vi "DAQmx Create Virtual Channel (CI Frequency).vi"(0 "task in":refnum<class "Session Factory.lvclass">, 1 "maximum value":dbl=100.0 format="%0.6f", 2 "minimum value":dbl=2.0 format="%0.6f", 3 "measurement method":i32(ring)=10105 items=["Low Frequency with 1 Counter"=10105, "High Frequency with 2 Counters"=10157, "Large Range with 2 Counters"=10205, "Dynamic Averaging"=16065], 5 "counter":tag, 6 "divisor":u32=4, 7 "name to assign":string, 9 "units":i32(ring)=10373 items=["Hz"=10373, "Ticks"=10304, "From Custom Scale"=10065], 11 "error in":errorcluster, 12 "custom scale name":tag, 13 "starting edge":i32(ring)=10280 items=["Rising"=10280, "Falling"=10171], 14 "measurement time":dbl=0.001 format="%0.6f") -> (4 "task out":refnum<class "Session Factory.lvclass">, 15 "error out":errorcluster)   [LabVIEW 2021, in "Session Management niDAQmx.lvlib" / "Session Factory.lvclass"]
doc: "Creates a channel to measure the frequency of a digital signal. With the exception of devices that support multi-counter tasks, you can create only one counter input channel at a time with this VI because a task can contain only one counter input channel. To read from multiple counters simultaneously, use a separate task for each counter. Connect the input signal to the default input terminal of the counter unless you select a different input terminal."
uses:
  Session Factory.lvclass
  NI_DAQmx_client/RPC Messages/nidaqmx_grpc_CreateCIFreqChanRequest.ctl
  NI_DAQmx_client/RPC Messages/nidevice_grpc_Session.ctl
  NI_DAQmx_client/RPC Messages/nidevice_grpc_Session_session/nidevice_grpc_Session_session.lvclass
  NI_DAQmx_client/RPC Messages/nidaqmx_grpc_CreateCIFreqChanRequest_units_enum/nidaqmx_grpc_CreateCIFreqChanRequest_units_enum.lvclass
  NI_DAQmx_client/RPC Messages/nidaqmx_grpc_CreateCIFreqChanRequest_edge_enum/nidaqmx_grpc_CreateCIFreqChanRequest_edge_enum.lvclass
  NI_DAQmx_client/RPC Messages/nidaqmx_grpc_CreateCIFreqChanRequest_meas_method_enum/nidaqmx_grpc_CreateCIFreqChanRequest_meas_method_enum.lvclass
  Session Factory.lvclass/Session Factory.ctl
  NI_DAQmx_client/RPC Messages/nidaqmx_grpc_CounterFrequencyMethod.ctl
  NI_DAQmx_client/RPC Messages/nidaqmx_grpc_CreateCIFreqChanRequest_meas_method_enum/nidaqmx_grpc_CreateCIFreqChanRequest_meas_method_enum.lvclass/nidaqmx_grpc_CreateCIFreqChanRequest_meas_method_enum.ctl
  NI_DAQmx_client/RPC Messages/nidaqmx_grpc_FrequencyUnits3.ctl
  NI_DAQmx_client/RPC Messages/nidaqmx_grpc_CreateCIFreqChanRequest_units_enum/nidaqmx_grpc_CreateCIFreqChanRequest_units_enum.lvclass/nidaqmx_grpc_CreateCIFreqChanRequest_units_enum.ctl
  NI_DAQmx_client/RPC Messages/nidaqmx_grpc_Edge1.ctl
  NI_DAQmx_client/RPC Messages/nidaqmx_grpc_CreateCIFreqChanRequest_edge_enum/nidaqmx_grpc_CreateCIFreqChanRequest_edge_enum.lvclass/nidaqmx_grpc_CreateCIFreqChanRequest_edge_enum.ctl
  NI_DAQmx_client/NI_DAQmx_client.lvlib
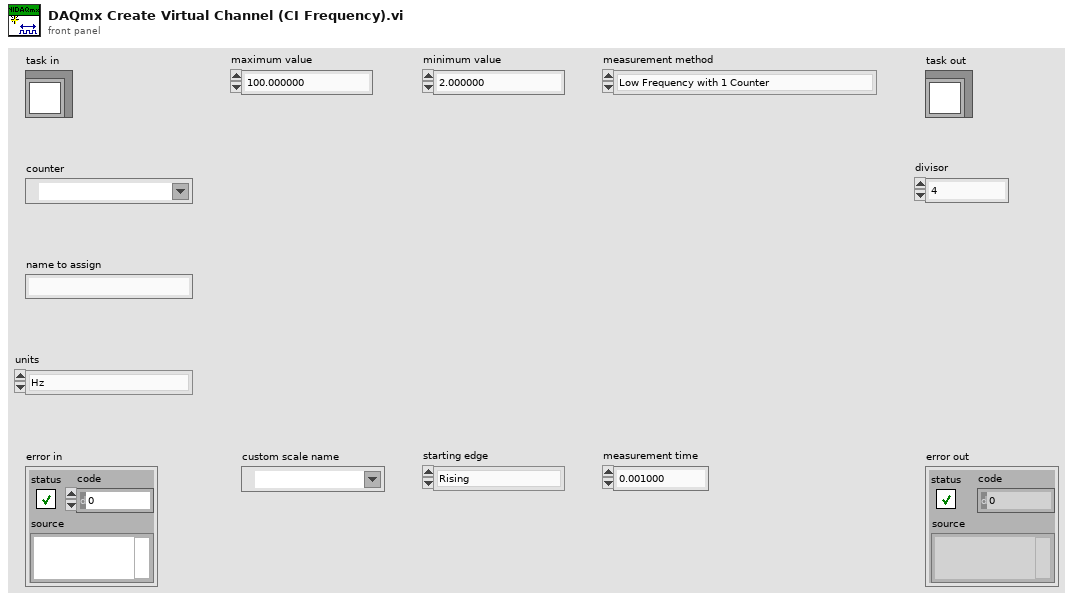
[diagram p1: front panel]
types:
  T1 = typedef "NI_DAQmx_client.lvlib/nidaqmx_grpc_CreateCIFreqChanRequest.ctl" = cluster{"task":T2, "counter":string, "name_to_assign_to_channel":string, "min_val":dbl, "max_val":dbl, "nidaqmx_grpc_CreateCIFreqChanRequest_units_enum":refnum<class "nidaqmx_grpc_CreateCIFreqChanRequest_units_enum.lvclass">, "nidaqmx_grpc_CreateCIFreqChanRequest_edge_enum":refnum<class "nidaqmx_grpc_CreateCIFreqChanRequest_edge_enum.lvclass">, "nidaqmx_grpc_CreateCIFreqChanRequest_meas_method_enum":refnum<class "nidaqmx_grpc_CreateCIFreqChanRequest_meas_method_enum.lvclass">, "meas_time":dbl, "divisor":u32, "custom_scale_name":string}
  T2 = typedef "NI_DAQmx_client.lvlib/nidevice_grpc_Session.ctl" = cluster{"nidevice_grpc_Session_session":refnum<class "nidevice_grpc_Session_session.lvclass">}
  T3 = typedef "NI_DAQmx_client.lvlib/nidaqmx_grpc_Edge1.ctl" = enum32{"EDGE1_UNSPECIFIED", "EDGE1_RISING", "EDGE1_FALLING"}
  T4 = typedef "NI_DAQmx_client.lvlib/nidaqmx_grpc_FrequencyUnits3.ctl" = enum32{"FREQUENCY_UNITS3_UNSPECIFIED", "FREQUENCY_UNITS3_HZ", "FREQUENCY_UNITS3_TICKS", "FREQUENCY_UNITS3_FROM_CUSTOM_SCALE"}
  T5 = typedef "NI_DAQmx_client.lvlib/nidaqmx_grpc_CounterFrequencyMethod.ctl" = enum32{"COUNTER_FREQUENCY_METHOD_UNSPECIFIED", "COUNTER_FREQUENCY_METHOD_LOW_FREQ_1_CTR", "COUNTER_FREQUENCY_METHOD_HIGH_FREQ_2_CTR", "COUNTER_FREQUENCY_METHOD_LARGE_RNG_2_CTR", "COUNTER_FREQUENCY_METHOD_DYN_AVG"}
  T6 = typedef "grpc-lvsupport-release.lvlib/grpcId.ctl" = u64
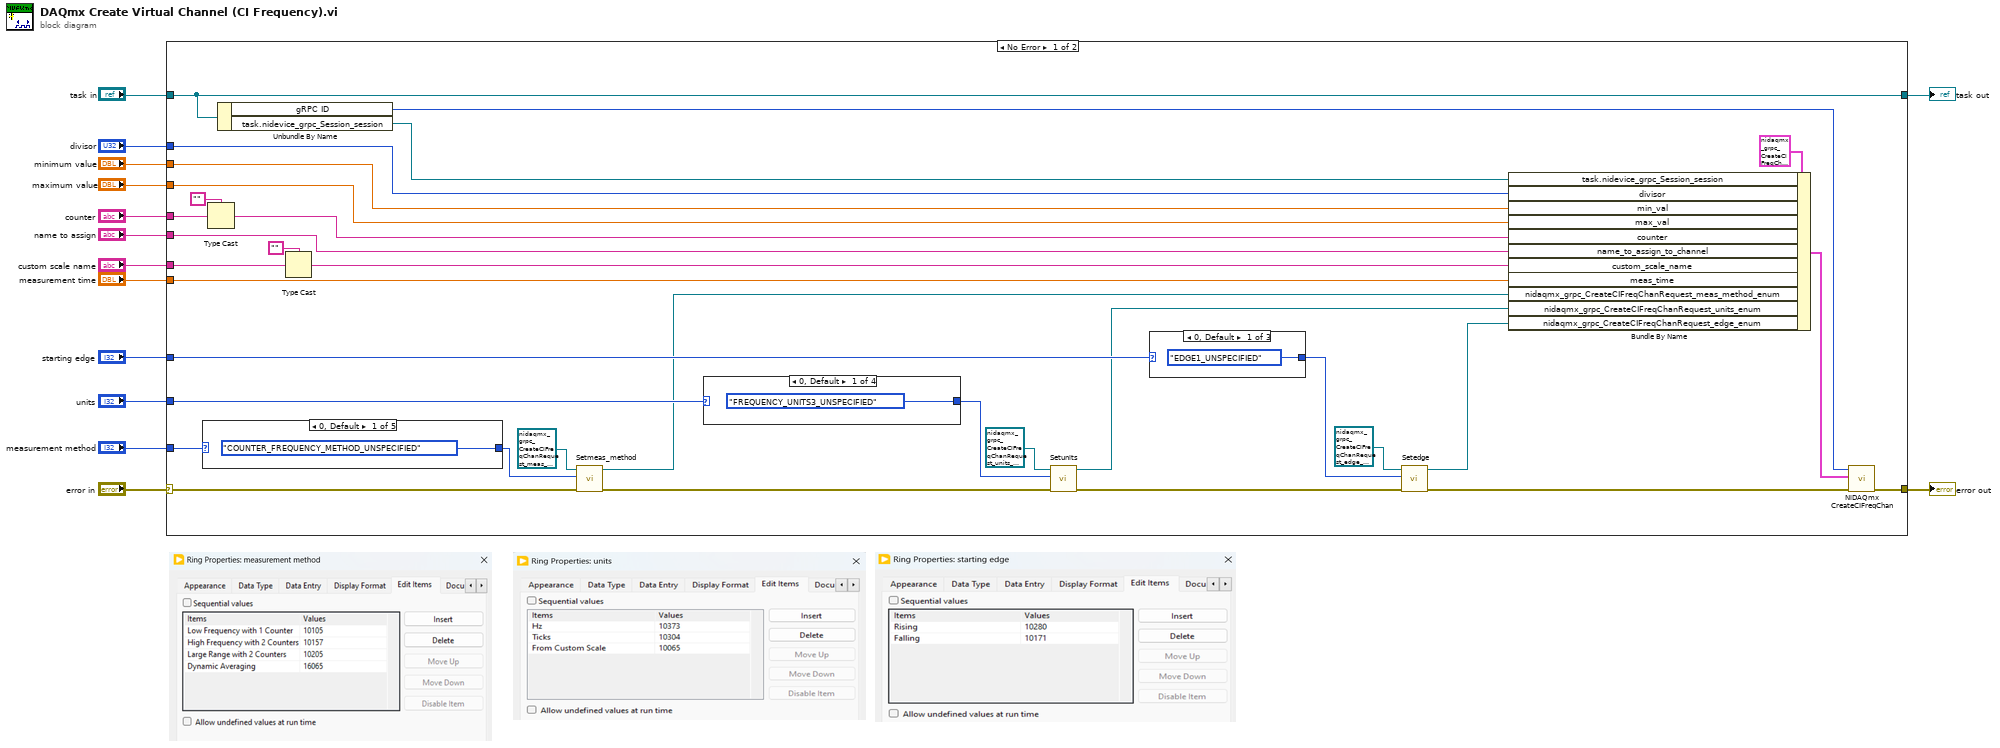
[diagram p0: block diagram]
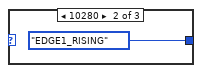
[diagram p2: hidden frame]
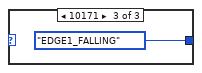
[diagram p3: hidden frame]
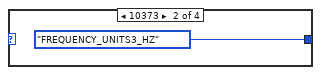
[diagram p4: hidden frame]
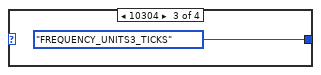
[diagram p5: hidden frame]
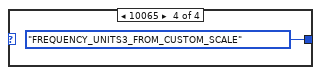
[diagram p6: hidden frame]
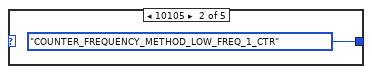
[diagram p7: hidden frame]
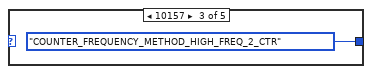
[diagram p8: hidden frame]
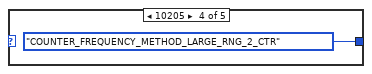
[diagram p9: hidden frame]
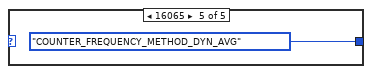
[diagram p10: hidden frame]
diagram:
  n1 = case shown="No Error" "error in" {
    selector: "error in" -> [w40 w61]
    tunnel: [w47 w61] -> w13
    tunnel: "task in" -> [w46 w60]
    tunnel: [w46 w60] -> w11
    tunnel: "divisor" -> [w41 _]
    tunnel: "measurement method" -> [w38 _]
    tunnel: "minimum value" -> [w16 _]
    tunnel: "maximum value" -> [w15 _]
    tunnel: "counter" -> [w18 _]
    tunnel: "name to assign" -> [w20 _]
    tunnel: "units" -> [w34 _]
    tunnel: "custom scale name" -> [w23 _]
    tunnel: "starting edge" -> [w30 _]
    tunnel: "measurement time" -> [w24 _]
    frame No Error {
      n2 = case shown="0, Default" w38 {
        tunnel: [nidaqmx_grpc_CounterFrequencyMethod."COUNTER_FREQUENCY_METHOD_UNSPECIFIED" ("Set_Val") nidaqmx_grpc_CounterFrequencyMethod."COUNTER_FREQUENCY_METHOD_LOW_FREQ_1_CTR" ("Set_Val") nidaqmx_grpc_CounterFrequencyMethod."COUNTER_FREQUENCY_METHOD_HIGH_FREQ_2_CTR" ("Set_Val") nidaqmx_grpc_CounterFrequencyMethod."COUNTER_FREQUENCY_METHOD_LARGE_RNG_2_CTR" ("Set_Val") nidaqmx_grpc_CounterFrequencyMethod."COUNTER_FREQUENCY_METHOD_DYN_AVG" ("Set_Val")] -> w37
        frame 0, Default {
        }
        frame 10105 {
        }
        frame 10157 {
        }
        frame 10205 {
        }
        frame 16065 {
        }
      }
      n3 = Type Cast(type="", x=w18) -> (*(type *) &x=w17:string)
      n4 = Unbundle By Name(w46) -> ("gRPC ID"=w45:T6, "task.nidevice_grpc_Session_session"=w43:refnum<class "nidevice_grpc_Session_session.lvclass">)
      n5 = Type Cast(type="", x=w23) -> (*(type *) &x=w21:string)
      n6 = call "Setmeas_method.vi"("error in (no error)"=w40, "Set_Val"=w37, "OneOfTemplate in"=refnum<class "nidaqmx_grpc_CreateCIFreqChanRequest_meas_method_enum.lvclass"> refnum) -> ("error out"=w36:errorcluster, "OneOfTemplate out"=w27:refnum<class "nidaqmx_grpc_CreateCIFreqChanRequest_meas_method_enum.lvclass">)  [unwired: 7 in]
      n7 = case shown="0, Default" w34 {
        tunnel: [nidaqmx_grpc_FrequencyUnits3."FREQUENCY_UNITS3_UNSPECIFIED" ("Set_Val") nidaqmx_grpc_FrequencyUnits3."FREQUENCY_UNITS3_HZ" ("Set_Val") nidaqmx_grpc_FrequencyUnits3."FREQUENCY_UNITS3_TICKS" ("Set_Val") nidaqmx_grpc_FrequencyUnits3."FREQUENCY_UNITS3_FROM_CUSTOM_SCALE" ("Set_Val")] -> w33
        frame 0, Default {
        }
        frame 10373 {
        }
        frame 10304 {
        }
        frame 10065 {
        }
      }
      n8 = call "Setunits.vi"("error in (no error)"=w36, "Set_Val"=w33, "OneOfTemplate in"=refnum<class "nidaqmx_grpc_CreateCIFreqChanRequest_units_enum.lvclass"> refnum) -> ("error out"=w32:errorcluster, "OneOfTemplate out"=w26:refnum<class "nidaqmx_grpc_CreateCIFreqChanRequest_units_enum.lvclass">)  [unwired: 7 in]
      n9 = case shown="0, Default" w30 {
        tunnel: [nidaqmx_grpc_Edge1."EDGE1_UNSPECIFIED" ("Set_Val") nidaqmx_grpc_Edge1."EDGE1_RISING" ("Set_Val") nidaqmx_grpc_Edge1."EDGE1_FALLING" ("Set_Val")] -> w29
        frame 0, Default {
        }
        frame 10280 {
        }
        frame 10171 {
        }
      }
      n10 = call "Setedge.vi"("error in (no error)"=w32, "Set_Val"=w29, "OneOfTemplate in"=refnum<class "nidaqmx_grpc_CreateCIFreqChanRequest_edge_enum.lvclass"> refnum) -> ("error out"=w31:errorcluster, "OneOfTemplate out"=w25:refnum<class "nidaqmx_grpc_CreateCIFreqChanRequest_edge_enum.lvclass">)  [unwired: 7 in]
      n11 = Bundle By Name(cluster=T1 {"task"={"nidevice_grpc_Session_session"=refnum}, "counter"="", "name_to_assign_to_channel"="", "min_val"=0.0, "max_val"=0.0, "nidaqmx_grpc_CreateCIFreqChanRequest_units_enum"=refnum, "nidaqmx_grpc_CreateCIFreqChanRequest_edge_enum"=refnum, "nidaqmx_grpc_CreateCIFreqChanRequest_meas_method_enum"=refnum, "meas_time"=0.0, "divisor"=0, "custom_scale_name"=""} ("Request Data"), "task.nidevice_grpc_Session_session"=w43, "divisor"=w41, "min_val"=w16, "max_val"=w15, "counter"=w17, "name_to_assign_to_channel"=w20, "custom_scale_name"=w21, "meas_time"=w24, "nidaqmx_grpc_CreateCIFreqChanRequest_meas_method_enum"=w27, "nidaqmx_grpc_CreateCIFreqChanRequest_units_enum"=w26, "nidaqmx_grpc_CreateCIFreqChanRequest_edge_enum"=w25) -> (w42:T1)
      n12 = call "NiDAQmx CreateCIFreqChan.vi"("error in"=w31, "Request Data"=w42, "gRPC ID"=w45) -> ("error out"=w47:errorcluster)  [unwired: 6 in, 2 out]
    }
    frame Error {
    }
  }
  "error out" <- w13
  "task out" <- w11
